vi "TempStatus.vi"(0 "VisaCluster":T2, 11 "error in (no error)":errorcluster) -> (4 "VisaCluster":T2, 8 "Answer":string, 10 "Temp_Unit":T1, 15 "error out":errorcluster)   [LabVIEW 2014, in "FH 55.lvlib"]
doc: "Dieses VI gibt die aktuellen Messwerte der Temperatur zurück.\n\nThis VI returns the current values of the temperature."
uses:
  FH 55.lvlib
  TypeDef/VisaCluster.ctl
  TypeDef/Temp_Unit.ctl
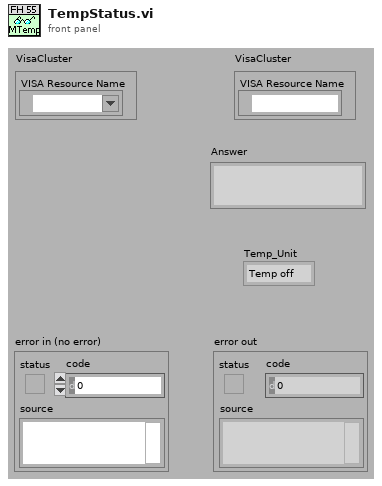
[diagram p1: front panel]
types:
  T1 = typedef "FH 55.lvlib/Temp_Unit.ctl" = enum16{"Temp off", "Celsius", "Fahrenheit"}
  T2 = typedef "FH 55.lvlib/VisaCluster.ctl" = cluster{"VISA Resource Name":refnum<visa-resource-name>}
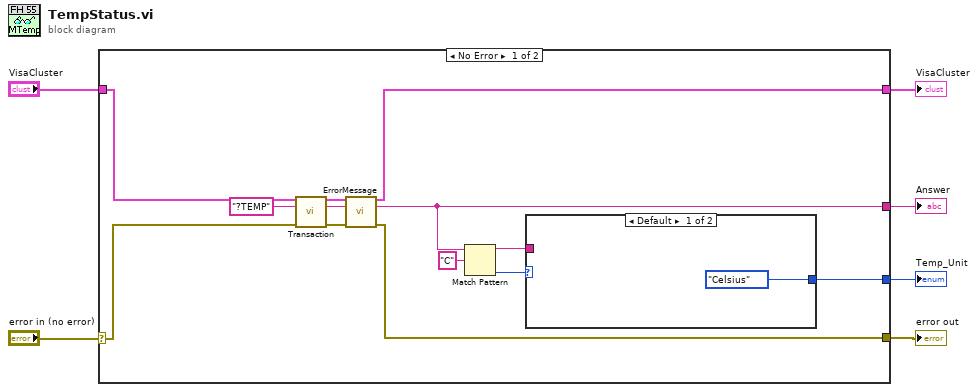
[diagram p0: block diagram]
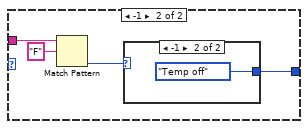
[diagram p2: hidden frame]
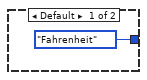
[diagram p3: hidden frame]
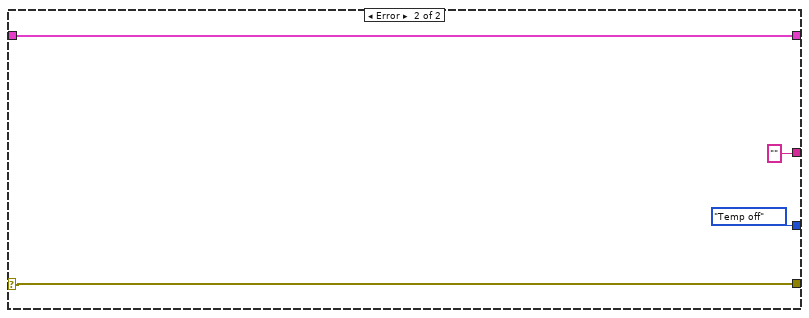
[diagram p4: hidden frame]
diagram:
  n1 = case shown="No Error" "error in (no error)" {
    selector: "error in (no error)" -> [w17 w28]
    tunnel: "VisaCluster" -> [w18 w30]
    tunnel: [w13 w30] -> w4
    tunnel: [w11 w28] -> w3
    tunnel: [w10 ""] -> w2
    tunnel: [w16 Temp_Unit."Temp off" ("Temp_Unit")] -> w1
    frame No Error {
      n2 = call "Transaction.vi"("VisaCluster"=w18, "Command"="?TEMP", "error in (no error)"=w17) -> ("VisaCluster"=w14:T2, "Answer"=w15:string, "error out"=w12:errorcluster)  [unwired: 9 in, 1 out]
      n3 = call "ErrorMessage.vi"("VisaCluster"=w14, "Message In"=w15, "error in (no error)"=w12) -> ("VisaCluster"=w13:T2, "Message Out"=w10:string, "error out"=w11:errorcluster)  [unwired: 10 in]
      n4 = Match Pattern(string=w10, regular expression="C") -> (before substring=w7:string, offset past match=w8:i32)  [unwired: 1 in, 2 out]
      n5 = case shown="Default" w8 {
        tunnel: [Temp_Unit."Celsius" ("Temp_Unit") w21] -> w16
        tunnel: w7 -> [_ w24]
        frame Default {
        }
        frame -1 {
          n6 = Match Pattern(string=w24, regular expression="F") -> (offset past match=w22:i32)  [unwired: 1 in, 3 out]
          n7 = case shown="-1" w22 {
            tunnel: [Temp_Unit."Fahrenheit" ("Temp_Unit") Temp_Unit."Temp off" ("Temp_Unit")] -> w21
            frame Default {
            }
            frame -1 {
            }
          }
        }
      }
    }
    frame Error {
    }
  }
  "error out" <- w3
  "Answer" <- w2
  "VisaCluster" <- w4
  "Temp_Unit" <- w1
